vi "Position Mission Method String.vi"(8 "error in (no error)":errorcluster, 10 "Title String":refnum<vi>, 11 "Mission Method Ref":refnum<vi>) -> (0 "error out":errorcluster)   [LabVIEW 2014]
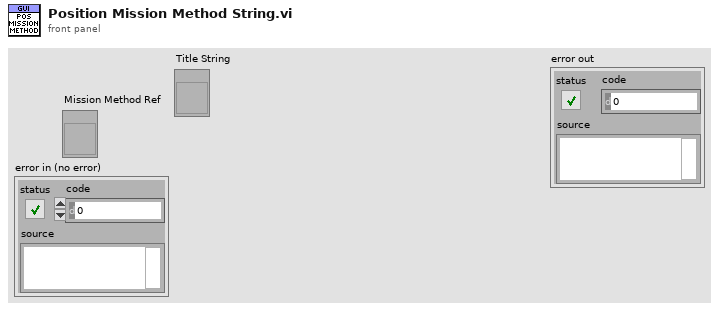
[diagram p1: front panel]
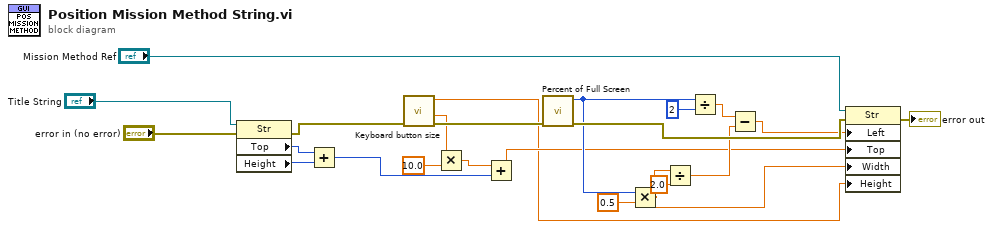
[diagram p0: block diagram]
diagram:
  n1 = property class="Str"(reference="Title String", error in="error in (no error)") -> (error out=w8:errorcluster, "Top"=w10:i32, "Height"=w9:u32)  [unwired: 1 out]
  n2 = Add(x=w10, y=w9) -> (x+y=w6:u32)
  n3 = call "Keyboard button size.vi"("error in (no error)"=w8) -> ("error out"=w7:errorcluster, "Key Spacing"=w3:dbl, "Key Height"=w1:dbl)  [unwired: 7 in, 1 out]
  n4 = Multiply(x=w3, y=10.0) -> (x*y=w4:dbl)
  n5 = Add(x=w4, y=w6) -> (x+y=w5:dbl)
  n6 = call "Percent of Full Screen.vi"("error in (no error)"=w7) -> ("error out"=w21:errorcluster, "Right"=w18:i16)  [unwired: 8 in, 1 out]
  n7 = Multiply(x=w18, y=0.5) -> (x*y=w15:dbl)
  n8 = Divide(x=w15, y=2.0) -> (x/y=w13:dbl)
  n9 = Divide(x=w18, y=i16 2) -> (x/y=w22:dbl)
  n10 = Subtract(x=w22, y=w13) -> (x-y=w20:dbl)
  n11 = property class="Str"(reference="Mission Method Ref", error in=w21, "Left"=w20, "Top"=w5, "Width"=w15, "Height"=w1) -> (error out=→"error out":errorcluster)  [unwired: 1 out]
